vi "Get_script_body.vi"(11 "Byte Stream File in":refnum<file>) -> (1 "Script Body":string[](array[string]), 2 "Full Text":string, 3 "File Path Out":path)   [LabVIEW 2017, in "labview-standard-library.lvlib"]
uses:
  labview-standard-library.lvlib
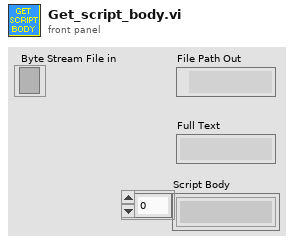
[diagram p1: front panel]
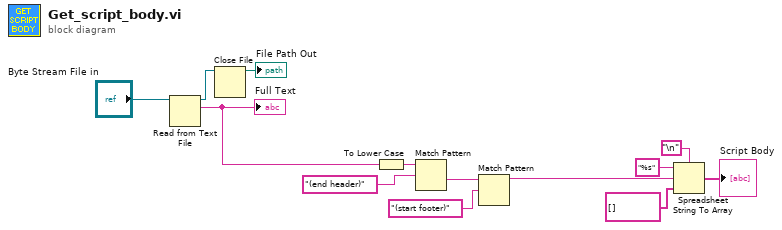
[diagram p0: block diagram]
diagram:
  n1 = Read from Text File(file (use dialog)="Byte Stream File in") -> (refnum out=w7:refnum<file>, text=w13:string)  [unwired: 3 in, 2 out]
  "Full Text" <- w13
  n2 = Close File(refnum=w7) -> (path=→"File Path Out":path)  [unwired: 1 in, 1 out]
  n3 = To Lower Case(string=w13) -> (all lower case string=w8:string)
  n4 = Match Pattern(string=w8, regular expression="(end header)") -> (after substring=w11:string)  [unwired: 1 in, 3 out]
  n5 = Match Pattern(string=w11, regular expression="(start footer)") -> (before substring=w2:string)  [unwired: 1 in, 3 out]
  n6 = Spreadsheet String To Array(delimiter (Tab)="\n", format string="%s", spreadsheet string=w2, array type (2D Dbl)=string[] [] ("appended array")) -> (array=→"Script Body":string[])
